vi "Enqueue an Item to Queue.vi"(7 "Add to Queue? (T)":bool=TRUE, 8 "Error In":errorcluster, 9 "Data (Optional)":variant, 10 "Item to Add":string, 11 "Queue Ref In":refnum<queue>) -> (0 "Error Out":errorcluster, 3 "Queue Ref Out":refnum<queue>)   [LabVIEW 2016, in "SLL QSM.lvlib"]
doc: "Adds an item to the Queue based on the input boolean flag - \"Add to Queue?\"."
uses:
  SLL QSM.lvlib
  Typedefs/Queue Type.ctl
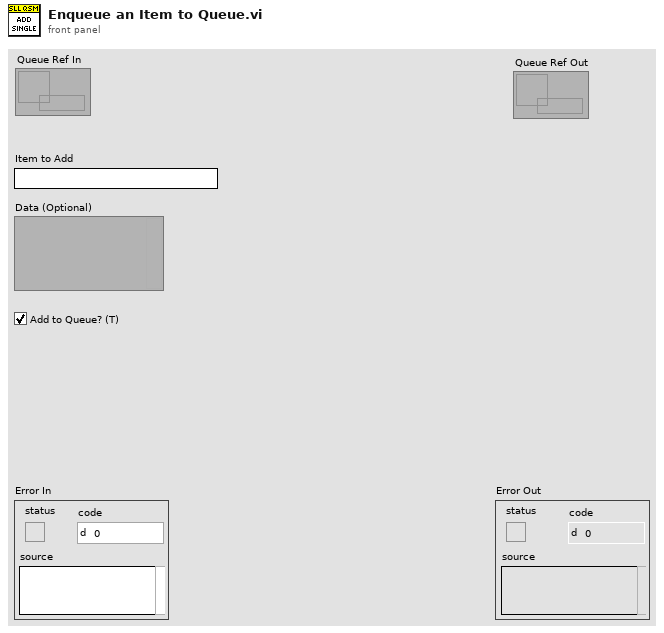
[diagram p1: front panel]
types:
  T1 = typedef "SLL QSM.lvlib/Queue Type.ctl" = cluster{"State":string, "Data":variant}
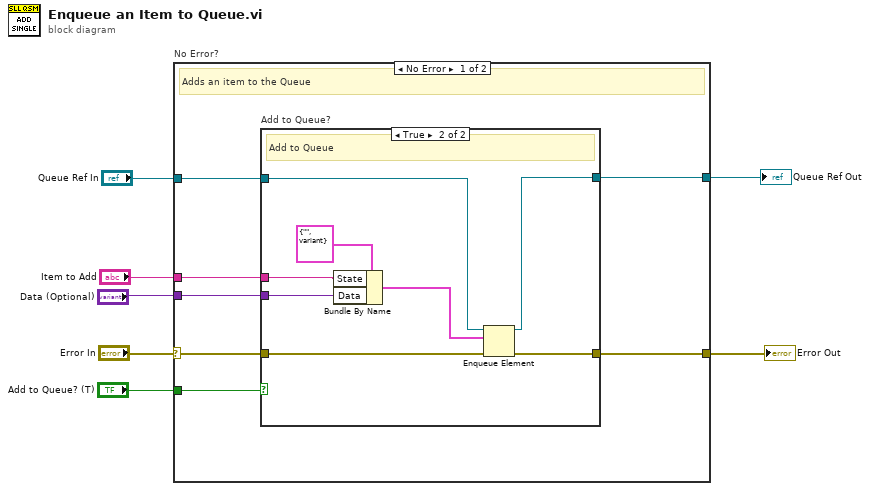
[diagram p0: block diagram]
diagram:
  n1 = case "No Error?" shown="No Error" "Error In" {
    selector: "Error In" -> [w12 w26]
    tunnel: [w14 w26] -> w7
    tunnel: "Item to Add" -> [w13 _]
    tunnel: "Add to Queue? (T)" -> [w11 _]
    tunnel: "Data (Optional)" -> [w10 _]
    tunnel: "Queue Ref In" -> [w9 w25]
    tunnel: [w8 w25] -> w1
    frame No Error {
      # "Adds an item to the Queue"
      n2 = case "Add to Queue?" shown="True" w11 {
        tunnel: w12 -> [w16 w18]
        tunnel: [w16 w24] -> w14
        tunnel: w13 -> [_ w22]
        tunnel: w10 -> [_ w20]
        tunnel: w9 -> [w15 w19]
        tunnel: [w15 w17] -> w8
        frame False {
          # "Skip Adding to Queue"
        }
        frame True {
          # "Add to Queue"
          n3 = Bundle By Name(cluster=T1 {"State"="", "Data"=variant} ("Queue Type"), "State"=w22, "Data"=w20) -> (w21:T1)
          n4 = Enqueue Element(queue=w19, element=w21, error in (no error)=w18) -> (queue out=w17:refnum<queue>, error out=w24:errorcluster)  [unwired: 1 in, 1 out]
        }
      }
    }
    frame Error {
    }
  }
  "Error Out" <- w7
  "Queue Ref Out" <- w1
